vi "Config Load Robot Globals.vi"(11 "refnum":T1) -> (3 "refnum 2":T1)   [LabVIEW 2012]
uses:
  <vilib>/Utility/config.llb/Config Data RefNum.ctl
  <vilib>/Utility/config.llb/Read Key (Double).vi
  Robot Global Data.vi
  <vilib>/Utility/config.llb/NI_LVConfig.lvlib
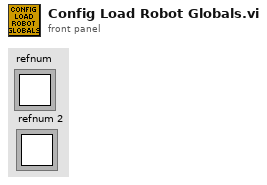
[diagram p1: front panel]
types:
  T1 = typedef "NI_LVConfig.lvlib/Config Data RefNum.ctl" = refnum<k1>
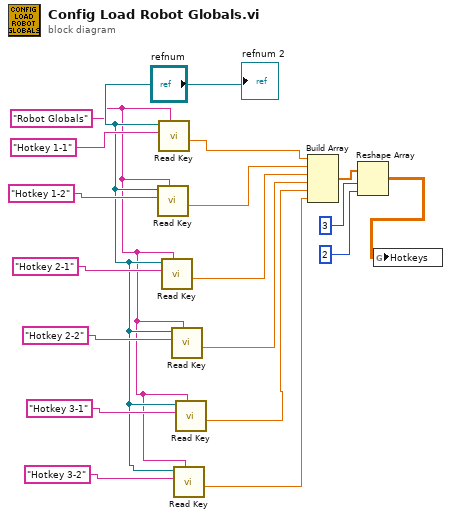
[diagram p0: block diagram]
diagram:
  w6 = "Robot Globals"
  n1 = call-poly <vilib>:"Read Key.vi"("section"=w6, "key"="Hotkey 1-2", "refnum"="refnum") -> ("value"=w15:dbl)  [unwired: 5 in, 3 out]
  n2 = call-poly <vilib>:"Read Key.vi"("section"=w6, "key"="Hotkey 1-1", "refnum"="refnum") -> ("value"=w18:dbl)  [unwired: 5 in, 3 out]
  n3 = call-poly <vilib>:"Read Key.vi"("section"=w6, "key"="Hotkey 2-1", "refnum"="refnum") -> ("value"=w13:dbl)  [unwired: 5 in, 3 out]
  n4 = call-poly <vilib>:"Read Key.vi"("section"=w6, "key"="Hotkey 2-2", "refnum"="refnum") -> ("value"=w10:dbl)  [unwired: 5 in, 3 out]
  n5 = call-poly <vilib>:"Read Key.vi"("section"=w6, "key"="Hotkey 3-2", "refnum"="refnum") -> ("value"=w5:dbl)  [unwired: 5 in, 3 out]
  n6 = call-poly <vilib>:"Read Key.vi"("section"=w6, "key"="Hotkey 3-1", "refnum"="refnum") -> ("value"=w9:dbl)  [unwired: 5 in, 3 out]
  n7 = Build Array(w18, w15, w13, w10, w9, w5) -> (w4:dbl[])
  n8 = Reshape Array(w4, 3, 2) -> (w3:dbl[][])
  n9 = global write "Robot Global Data.vi" "Hotkeys"(w3) -> ()
  "refnum 2" <- "refnum"
